vi "Tosca-Update Analysis.vi"(0 "Result":T1, 1 "MATLAB":refnum<notifier>, 2 "StimCon Element":T2, 5 "History":string[](array[string]), 7 "Result String":string, 9 "Rxn time":i32, 11 "error in (no error)":errorcluster, 12 "Analysis":T5, 13 "Control Refs":T11) -> (4 "Result thru":T1, 14 "Analysis out":T5, 15 "error out":errorcluster)   [LabVIEW 2020]
uses:
  Typedefs/Tosca-Trial Result Enum.ctl
  Typedefs/Tosca-Control Refs.ctl
  FSM Graph VIs/LV Source/FSM Editor/FSM Editor.xctl
  Typedefs/Tosca-Analysis State.ctl
  Typedefs/Tosca-Adaptation State.ctl
  Typedefs/Tosca-Adaptation Track State.ctl
  Typedefs/Tosca-Adaptation History Element.ctl
  Classes/Parameters/Histogram Data.ctl
  Classes/Parameters/Connect.ctl
  Typedefs/Tosca-SCL Element.ctl
  Typedefs/Tosca-Schedule Mode.ctl
  Typedefs/Tosca-Event Type.ctl
  Typedefs/Tosca-MATLAB Queue Data.ctl
  Classes/Parameters/Parameters.lvclass
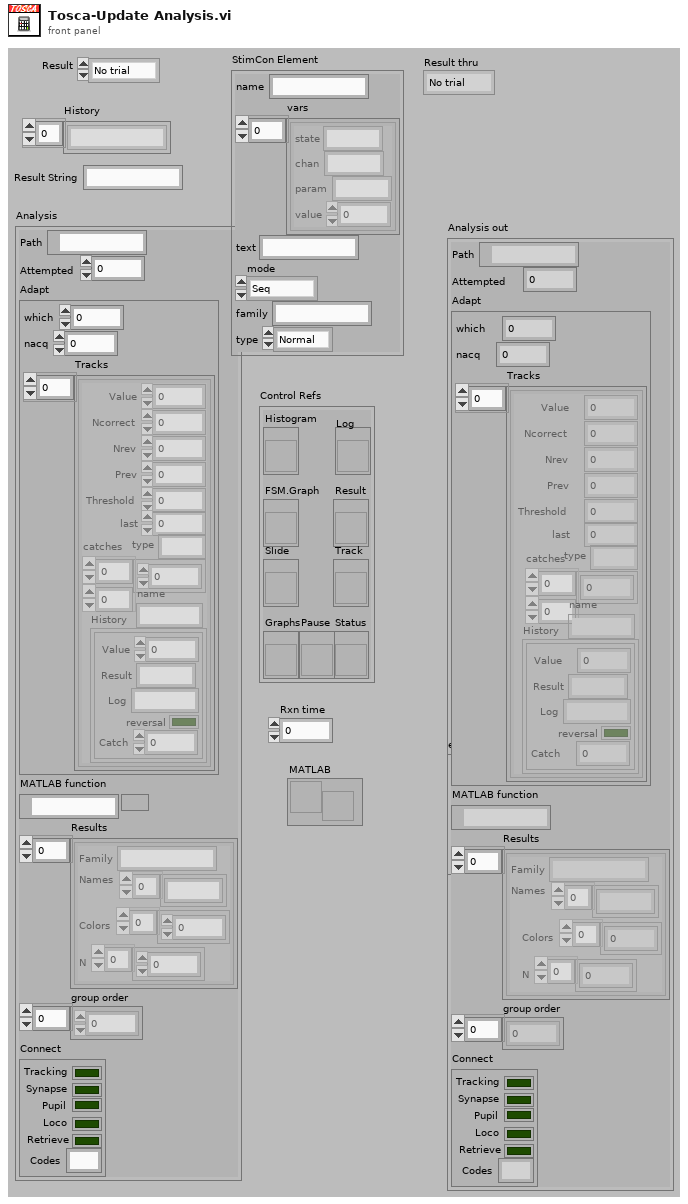
[diagram p1: front panel]
types:
  T1 = typedef "Tosca-Trial Result Enum.ctl" = enum16{"No trial", "Go", "No go", "Error", "Abort"}
  T2 = typedef "Tosca-SCL Element.ctl" = cluster{"name":string, "vars":cluster{"state":string, "chan":string, "param":string, "value":dbl}[], "text":string, "mode":T3, "family":string, "type":T4}
  T3 = typedef "Tosca-Schedule Mode.ctl" = enum16{"Seq", "CS+/CS-", "Adapt"}
  T4 = typedef "Tosca-Event Type.ctl" = enum16{"Normal", "CS+", "CS-"}
  T5 = typedef "Tosca-Analysis State.ctl" = cluster{"Path":path, "Attempted":i32, "Adapt":T6, "MATLAB function":path, "Results":T9[], "group order":i32[], "Connect":T10}
  T6 = typedef "Tosca-Adaptation State.ctl" = cluster{"which":i32, "nacq":i32, "Tracks":T7[]}
  T7 = typedef "Tosca-Adaptation Track State.ctl" = cluster{"Value":dbl, "Ncorrect":i32, "Nrev":i32, "Prev":dbl, "History":T8[], "Threshold":dbl, "last":i32, "type":string, "catches":dbl[][], "name":string}
  T8 = typedef "Tosca-Adaptation History Element.ctl" = cluster{"Value":dbl, "Result":string, "Log":string, "reversal":bool, "Catch":dbl}
  T9 = typedef "Parameters.lvclass/Histogram Data.ctl" = cluster{"Family":string, "Names":string[], "Colors":u32[], "N":i32[]}
  T10 = typedef "Parameters.lvclass/Connect.ctl" = cluster{"Tracking":bool, "Synapse":bool, "Pupil":bool, "Loco":bool, "Retrieve":bool, "Codes":string}
  T11 = typedef "Tosca-Control Refs.ctl" = cluster{"FSM.Graph":refnum<vi>, "Slide":refnum<vi>, "Result":refnum<vi>, "Histogram":refnum<vi>, "Graphs":refnum<vi>, "Track":refnum<vi>, "Log":refnum<vi>, "Status":refnum<vi>, "Pause":refnum<vi>}
  T12 = cluster{"MATLAB function":path, "file path out":path}
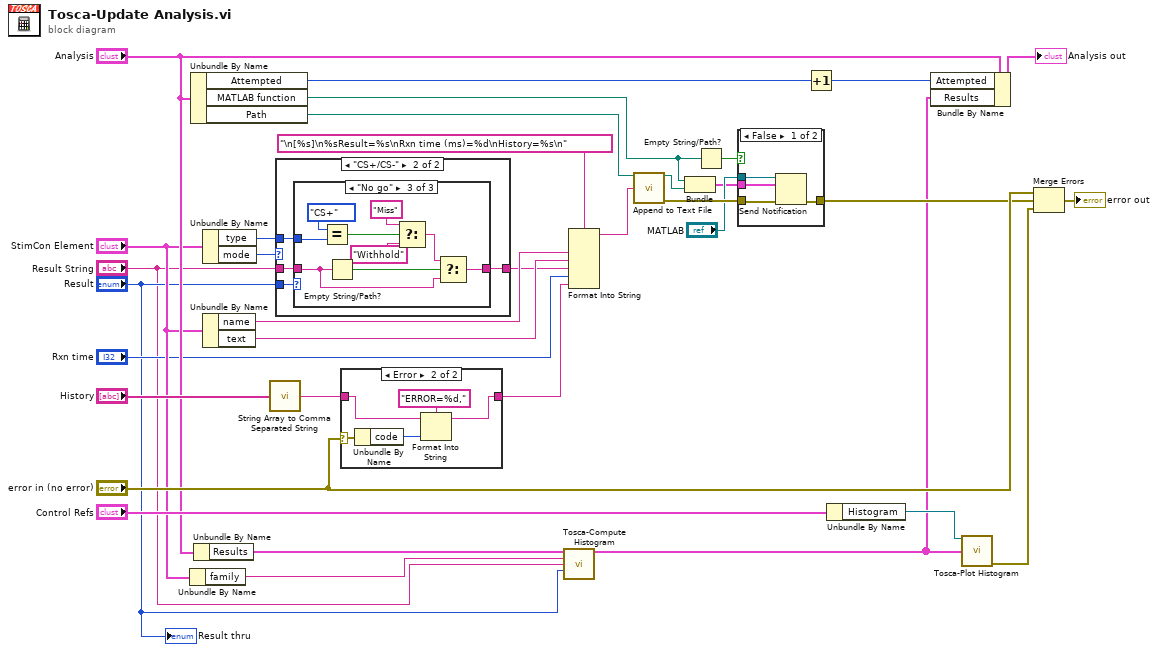
[diagram p0: block diagram]
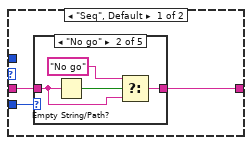
[diagram p2: hidden frame]
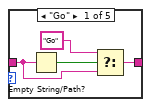
[diagram p3: hidden frame]
diagram:
  n1 = Unbundle By Name("StimCon Element") -> ("family"=w3:string)
  n2 = Unbundle By Name("Analysis") -> ("Attempted"=w31:i32, "MATLAB function"=w21:path, "Path"=w32:path)
  n3 = Unbundle By Name("Analysis") -> ("Results"=w4:T9[])
  n4 = Unbundle By Name("StimCon Element") -> ("type"=w9:T4, "mode"=w11:T3)
  n5 = Unbundle By Name("StimCon Element") -> ("name"=w14:string, "text"=w17:string)
  n6 = call "String Array to Comma Separated String.vi"("String Array"="History") -> ("comma separated string"=w25:string)
  n7 = case shown="\"CS+/CS-\"" w11 {
    tunnel: "Result String" -> [w37 w50]
    tunnel: [w36 w51] -> w10
    tunnel: w9 -> [_ w49]
    tunnel: "Result" -> [w35 w52]
    frame "Seq", Default {
      n8 = case shown="\"No go\"" w35 {
        tunnel: [w38 w42 w46 w47 w48] -> w36
        tunnel: w37 -> [w39 w43 w46 w47 w48]
        frame "Go" {
          n9 = Empty String/Path?(string/path=w39) -> (empty?=w41:bool)
          n10 = Select(t="Go", s=w41, f=w39) -> (s? t:f=w38:string)
        }
        frame "No go" {
          n11 = Empty String/Path?(string/path=w43) -> (empty?=w45:bool)
          n12 = Select(t="No go", s=w45, f=w43) -> (s? t:f=w42:string)
        }
        frame "Abort", Default {
        }
        frame "Error" {
        }
        frame "No trial" {
        }
      }
    }
    frame "CS+/CS-" {
      n13 = case shown="\"No go\"" w52 {
        tunnel: [w53 w54 w56] -> w51
        tunnel: w50 -> [w53 w54 w55]
        tunnel: w49 -> [_ _ w61]
        frame "No trial", Default {
        }
        frame "Go" {
        }
        frame "No go" {
          n14 = Equal?(x=Tosca-Event_Type."CS+", y=w61) -> (x = y?=w60:bool)
          n15 = Empty String/Path?(string/path=w55) -> (empty?=w57:bool)
          n16 = Select(t="Miss", s=w60, f="Withhold") -> (s? t:f=w58:string)
          n17 = Select(t=w58, s=w57, f=w55) -> (s? t:f=w56:string)
        }
      }
    }
  }
  n18 = case shown="Error" "error in (no error)" {
    selector: "error in (no error)" -> [_ w69]
    tunnel: w25 -> [w64 w67]
    tunnel: [w64 w66] -> w16
    frame No Error {
    }
    frame Error {
      n19 = Unbundle By Name(w69) -> ("code"=w68:i32)
      n20 = Format Into String(format string="ERROR=%d,", initial string=w67, w68) -> (resulting string=w66:string)  [unwired: 1 in, 1 out]
    }
  }
  n21 = call "Tosca-Compute Histogram.vi"("Results in"=w4, "family"=w3, "Result String"="Result String", "Result"="Result") -> ("Results out"=w6:T9[])  [unwired: 11 in]
  n22 = Format Into String(format string="\n[%s]\n%sResult=%s\nRxn time (ms)=%d\nHistory=%s\n", w14, w17, w10, "Rxn time", w16) -> (resulting string=w15:string)  [unwired: 2 in, 1 out]
  n23 = call "Append to Text File.vi"("file path"=w32, "text"=w15) -> ("file path out"=w20:path, "error out"=w24:errorcluster)  [unwired: 12 in]
  n24 = Bundle("MATLAB function"=w21, "file path out"=w20) -> (w19:T12)  [unwired: 1 in]
  n25 = Empty String/Path?(string/path=w21) -> (empty?=w23:bool)
  n26 = case shown="False" w23 {
    tunnel: w24 -> [w73 w74]
    tunnel: [w72 w74] -> w8
    tunnel: "MATLAB" -> [w71 _]
    tunnel: w19 -> [w70 _]
    frame False {
      n27 = Send Notification(notification=w70, notifier=w71, error in (no error)=w73) -> (error out=w72:errorcluster)  [unwired: 1 out]
    }
    frame True {
    }
  }
  n28 = Increment(x=w31) -> (x+1=w30:i32)
  n29 = Unbundle By Name("Control Refs") -> ("Histogram"=w29:refnum<vi>)
  n30 = Bundle By Name(cluster="Analysis", "Attempted"=w30, "Results"=w6) -> (→"Analysis out":T5)
  n31 = call "Tosca-Plot Histogram.vi"("Histogram"=w29, "Results"=w6) -> ("error out"=w7:errorcluster)  [unwired: 13 in]
  n32 = Merge Errors("error in (no error)", w8, w7) -> (→"error out":errorcluster)
  "Result thru" <- "Result"
